vi "cm_Level Color Current Write.vi"(4 "error in (no error)":errorcluster, 5 "Value":u32(colorbox)=6618880, 6 "Container State":T3, 7 "Display State In":T1={"Chan"=[], "First Drop?"=FALSE, "Notifier Name"="", "Refresh View"=FALSE, "Scale to Input Range"=FALSE, "Linear View"=FALSE, "Display"={"Current"=6618880, "Peak"=6618880}, "Property/Method"=enum."No Update", "Time Display Ref"=[]}) -> (0 "error out":errorcluster, 3 "Display State Out":T1={"Chan"=[], "First Drop?"=FALSE, "Notifier Name"="", "Refresh View"=FALSE, "Scale to Input Range"=FALSE, "Linear View"=FALSE, "Display"={"Current"=6618880, "Peak"=6618880}, "Property/Method"=enum."No Update", "Time Display Ref"=[]})   [LabVIEW 2012, in "Channel Monitor.xctl"]
doc: "Set the color of the current peak bar."
uses:
  Channel Monitor.xctl
  <vilib>/_xctls/Container State.ctl
  subVIs/cm_Channel Monitor State.ctl
  TypeDef/cm_Property_Method.ctl
  <vilib>/_xctls/XControlSupport.lvlib
panel:
  # "Replace the Value Control below with a Control of desired type.\nDo not remove this Control or the others from the connector pane.\nDo not change the connector pane pattern.\nThe Value control should always be the third terminal from top on the input side in the connector pane."
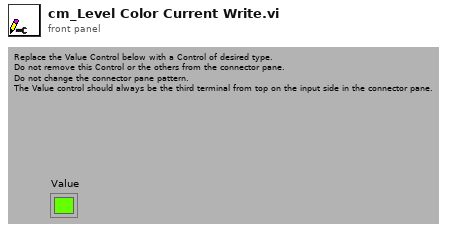
[diagram p1: front panel]
types:
  T1 = typedef "Channel Monitor.xctl/cm_Channel Monitor State.ctl" = cluster{"Chan":cluster{"ChanName":string, "Current":dbl, "Peak":dbl, "Input Range":dbl}[], "First Drop?":bool, "Notifier Name":string, "Refresh View":bool, "Scale to Input Range":bool, "Linear View":bool, "Display":cluster{"Current":u32, "Peak":u32}, "Property/Method":T2, "Time Display Ref":refnum<vi>[]}
  T2 = typedef "Channel Monitor.xctl/cm_Property_Method.ctl" = enum16{"No Update", "Color: Currrent", "Color: Peak", "Close Time Displays"}
  T3 = typedef "XControlSupport.lvlib/Container State.ctl" = cluster{"Indicator?":bool, "Run Mode?":bool, " Refnum":refnum<vi>}
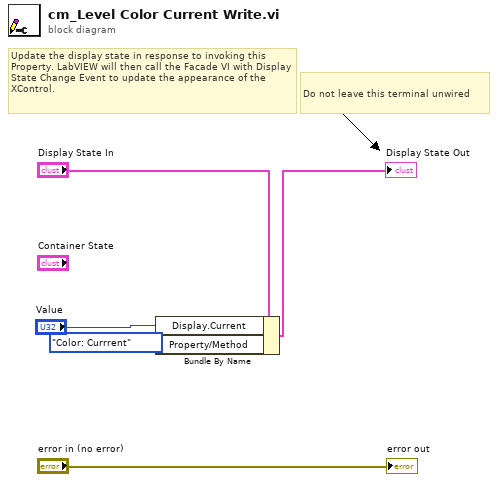
[diagram p0: block diagram]
diagram:
  # "Do not leave this terminal unwired"
  # "Update the display state in response to invoking this Property. LabVIEW will then call the Facade VI with Display State Change Event to update the appearance of the XControl."
  n1 = Bundle By Name(cluster="Display State In", "Display.Current"="Value", "Property/Method"=cm_Property_Method."Color: Currrent") -> (→"Display State Out":T1)
  "error out" <- "error in (no error)"
